vi "CFU_6p1_TEAM027.vi"() -> ()   [LabVIEW 2016]
panel:
  in  "Numeric":dbl
  out "Cr":dbl
  in  "Permiability Coefficent":dbl
  out "Days":dbl
  in  "Desired Concentration":dbl
  in  "Drug Concentration (Cd)":dbl
  in  "Volume":dbl
  in  "Area":dbl
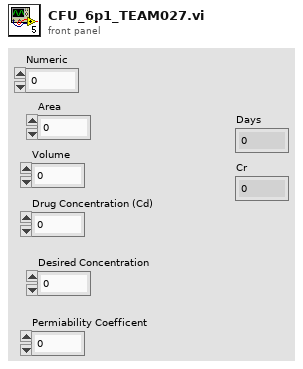
[diagram p1: front panel]
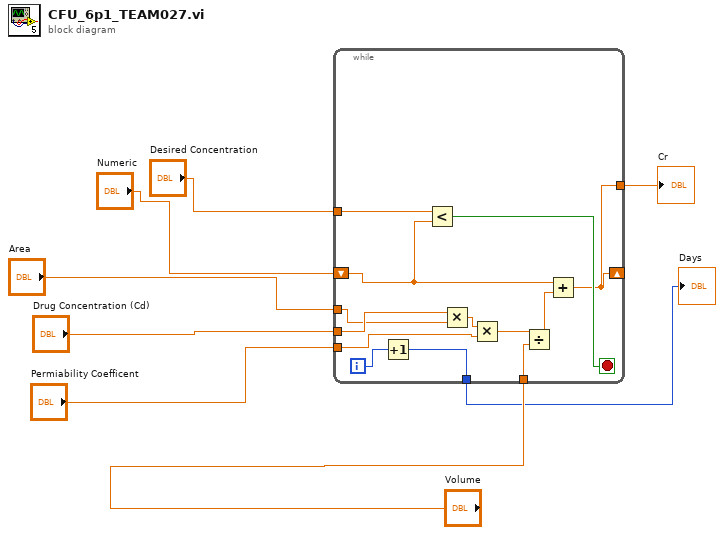
[diagram p0: block diagram]
diagram:
  n1 = while {
    shift-right: [w9] -> _
    shift-left: "Numeric" -> [w13]
    tunnel: "Drug Concentration (Cd)" -> [w19]
    tunnel: "Area" -> [w18]
    tunnel: "Volume" -> [w17]
    tunnel: "Desired Concentration" -> [w14]
    tunnel: [w11] -> w5
    tunnel: "Permiability Coefficent" -> [w10]
    tunnel: [w9] -> w2
    i -> [w21]
    stop <- w12 stop-if-true
    n2 = Increment(x=w21) -> (x+1=w11:i32)
    n3 = Less?(x=w14, y=w13) -> (x < y?=w12:bool)
    n4 = Multiply(x=w19, y=w18) -> (x*y=w20:dbl)
    n5 = Multiply(x=w20, y=w10) -> (x*y=w16:dbl)
    n6 = Divide(x=w16, y=w17) -> (x/y=w15:dbl)
    n7 = Add(x=w13, y=w15) -> (x+y=w9:dbl)
  }
  "Days" <- w5
  "Cr" <- w2
